vi "Renishaw-XL80_GetSignalStrength.vi"(8 "error in (no error)":errorcluster, 11 "Renishaw-XL80_EMU in":refnum<class "Renishaw-XL80_EMU.lvclass">) -> (0 "error out":errorcluster, 2 "Signal Strength":i16, 3 "Renishaw-XL80_EMU out":refnum<class "Renishaw-XL80_EMU.lvclass">)   [LabVIEW 2024, in "Renishaw-XL80_EMU.lvclass"]
doc: "This read only property returns the current signal strength of the ML10.\n\nDefinition\nHRESULTget_SignalStrength( [out, retval] short* pVal);\nParameters\npVal\nA variable that will be set to the signal strength of the ML10.\n\nComments\nThis property will return with an HRESULT of E_FAIL if the client has not previously connected to a DX10 by calling Connect.\n\nOtherwise the property will normally return an HRESULT of S_OK. However, it will return E_POINTER if the client supplies a null pointer for pVal.\n\nIf the ML10 is not responding then the signal strength will return the last known good value.\n\nThe signal strength is a value between 0 and 31, where 31 implies 100% signal strength. Note that it is customary to truncate any signal strength display meter at 26. So the user doesn't waste time trying to achieve signal strengths close to 100% which will have no benefit to measurement accuracy."
uses:
  Renishaw-XL80_EMU.lvclass
  <vilib>/numeric/Random Number (Range) I64.vi
  <vilib>/numeric/sub_Random U32.vi
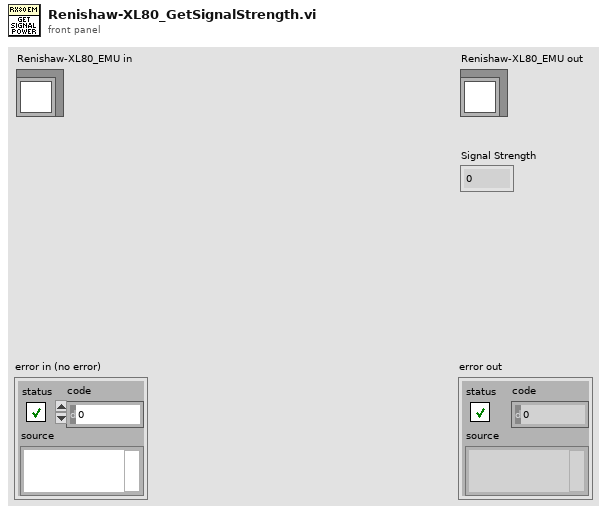
[diagram p1: front panel]
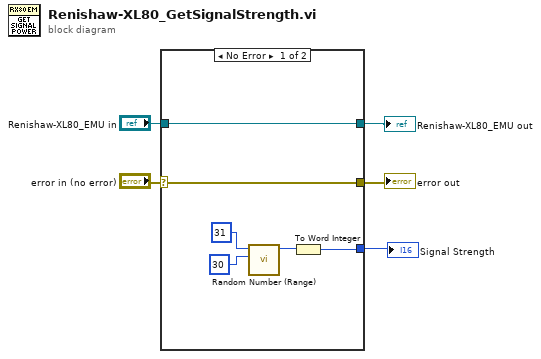
[diagram p0: block diagram]
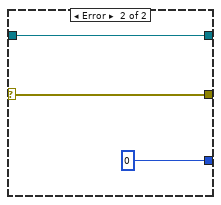
[diagram p2: hidden frame]
diagram:
  n1 = case shown="No Error" "error in (no error)" {
    selector: "error in (no error)" -> [w10 w13]
    tunnel: [w11 w14] -> w1
    tunnel: "Renishaw-XL80_EMU in" -> [w11 w14]
    tunnel: [w10 w13] -> w3
    tunnel: [w6 i16 0 ("GetAirTemp")] -> w2
    frame No Error {
      n2 = call-poly <vilib>:"Random Number (Range).vi"("lower bound (-100)"=i64 30 ("lower bound (0)"), "upper bound (100)"=i64 31) -> ("number"=w7:i64)  [unwired: 9 in]
      n3 = To Word Integer(number=w7) -> (16bit integer=w6:i16)
    }
    frame Error {
    }
  }
  "error out" <- w3
  "Renishaw-XL80_EMU out" <- w1
  "Signal Strength" <- w2
